vi "Query - Int64 - 2D.vi"(8 "error in":errorcluster, 10 "Query":string, 11 "Module ID":i32=-1) -> (0 "error out":errorcluster, 1 "Meta Data":variant, 2 "Return Data":i64[][](array[numeric]), 4 "Field Names":string[](array[string]))   [LabVIEW 2014, in "DB_CONNECTOR.lvlib"]
uses:
  DB_CONNECTOR.lvlib
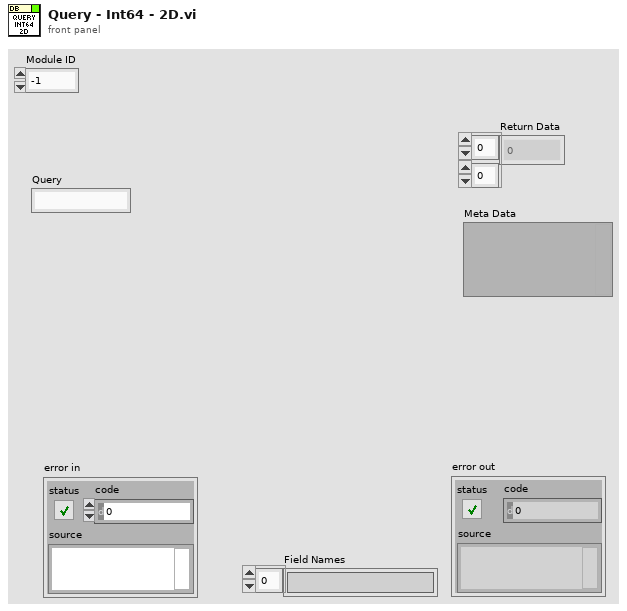
[diagram p1: front panel]
types:
  T1 = typedef "DB_CONNECTOR.lvlib/Query (Reply Payload)--cluster.ctl" = cluster{"Return Data":string[][], "Meta Data":variant, "Field Names":string[], "Query_error":errorcluster}
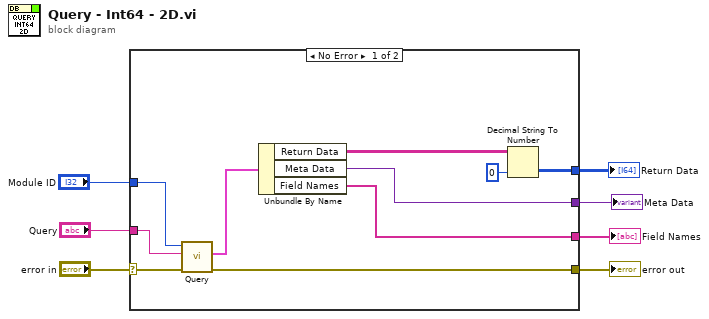
[diagram p0: block diagram]
diagram:
  n1 = case shown="No Error" "error in" {
    selector: "error in" -> [w17 w18]
    tunnel: [w12 w18] -> w6
    tunnel: "Query" -> [w15 _]
    tunnel: "Module ID" -> [w14 _]
    tunnel: [w11 _] -> w2
    tunnel: [w9 _] -> w3
    tunnel: [w8 _] -> w1
    frame No Error {
      n2 = call "Query.vi"("error in (no error)"=w17, "Query"=w15, "Module ID"=w14) -> ("error out"=w12:errorcluster, "Reply Payload"=w16:T1)  [unwired: 7 in]
      n3 = Unbundle By Name(w16) -> ("Return Data"=w13:string[][], "Meta Data"=w11:variant, "Field Names"=w8:string[])
      n4 = Decimal String To Number(string=w13, default (0L)=i64 0 ("default (0 I32)")) -> (number=w9:i64[][])  [unwired: 1 in, 1 out]
    }
    frame Error {
    }
  }
  "error out" <- w6
  "Return Data" <- w3
  "Meta Data" <- w2
  "Field Names" <- w1
